vi "field raster.vi"(0 "field size":dbl, 2 "field number":u32) -> (10 "Plot1":cluster{dbl[], dbl[]}, 11 "Plot2":cluster{dbl[], dbl[]}, 14 "current X":dbl, 15 "current Y":dbl, 17 "x mark":dbl[](array[numeric]), 18 "y mark":dbl[](array[numeric]))   [LabVIEW 2014]
uses:
  stage-controller-globals.vi
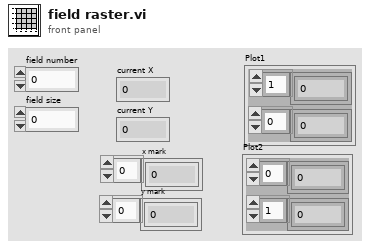
[diagram p1: front panel]
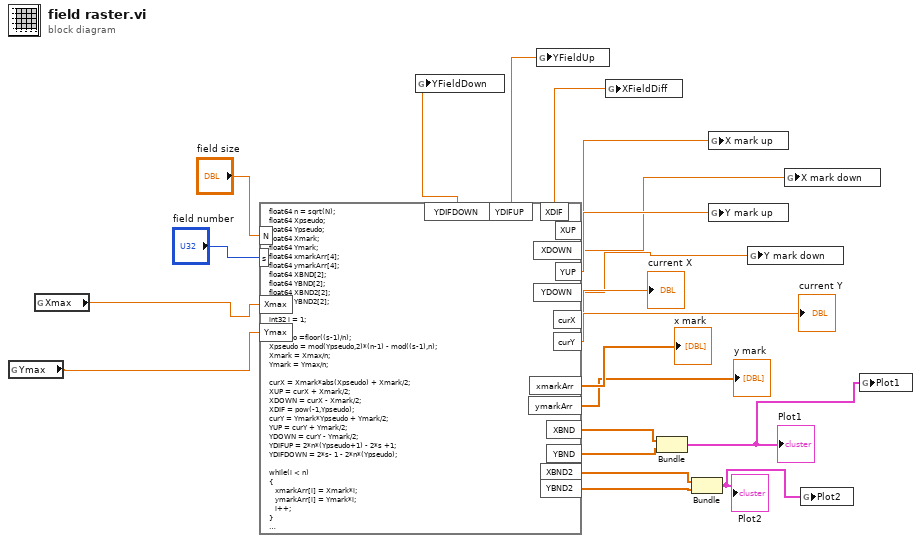
[diagram p0: block diagram]
diagram:
  n1 = global read "stage-controller-globals.vi" "Ymax"() -> (w10:dbl)
  n2 = global read "stage-controller-globals.vi" "Xmax"() -> (w11:dbl)
  n3 = formula code="float64 n = sqrt(N);\nfloat64 Xpseudo;\nfloat64 Ypseudo;\nfloat64 Xmark;\nfloat64 Ymark;\nfloat64 xmarkArr[4];\nfloat64 ymarkArr[4];\nfloat64 XBND[2];\nfloat64 YBND[2];\nfloat64 XBND2[2];\nfloat64 YBND2[2];\n\nint32 i = 1;\n\nYpseudo =floor((s-1)/n); \nXpseudo = mod(Ypseudo,2)*(n-1) - mod((s-1),n);\nXmark = Xmax/n;\nYmark = Ymax/n;\n\ncurX = Xmark*abs(Xpseudo) + Xmark/2;\nXUP = curX + Xmark/2;\nXDOWN = curX - Xmark/2;\nXDIF = pow(-1,Ypseudo);\ncurY = Ymark*Ypseudo + Ymark/2;\nYUP = curY + Ymark/2;\nYDOWN = curY - Ymark/2;\nYDIFUP = 2*n*(Ypseudo+1) - 2*s +1;\nYDIFDOWN = 2*s- 1 - 2*n*(Ypseudo);\n\nwhile(i < n)\n{\n   xmarkArr[i] = Xmark*i;\n   ymarkArr[i] = Ymark*i;\n   i++;\n}\n\ni = 0;\n\n XBND[i] = curX - Xmark/2;\nYBND[i] = curY - Ymark/2;\n i++;\nXBND[i] = curX + Xmark/2;\nYBND[i] = curY - Ymark/2;\n\ni=0;\n\nXBND2[i] = curX - Xmark/2;\nYBND2[i] =  curY + Ymark/2;\ni++;\nXBND2[i] = curX + Xmark/2;\nYBND2[i] =  curY + Ymark/2;\ni++;"("N"="field size", "s"="field number", "Xmax"=w11, "Ymax"=w10) -> ("curX"=→"current X":dbl, "curY"=→"current Y":dbl, "ymarkArr"=→"y mark":dbl[], "xmarkArr"=→"x mark":dbl[], "XUP"=w6:dbl, "YUP"=w7:dbl, "XBND"=w15:dbl[], "YBND"=w14:dbl[], "XBND2"=w13:dbl[], "YBND2"=w12:dbl[], "XDOWN"=w5:dbl, "YDOWN"=w4:dbl, "YDIFUP"=w3:dbl, "XDIF"=w2:dbl, "YDIFDOWN"=w1:dbl)
  n4 = global write "stage-controller-globals.vi" "YFieldDown"(w1) -> ()
  n5 = global write "stage-controller-globals.vi" "YFieldUp"(w3) -> ()
  n6 = global write "stage-controller-globals.vi" "XFieldDiff"(w2) -> ()
  n7 = Bundle(w15, w14) -> (w17:cluster{dbl[], dbl[]})  [unwired: 1 out]
  "Plot1" <- w17
  n8 = Bundle(w13, w12) -> (w16:cluster{dbl[], dbl[]})  [unwired: 1 out]
  "Plot2" <- w16
  n9 = global write "stage-controller-globals.vi" "X mark up"(w6) -> ()
  n10 = global write "stage-controller-globals.vi" "Y mark up"(w7) -> ()
  n11 = global write "stage-controller-globals.vi" "Y mark down"(w4) -> ()
  n12 = global write "stage-controller-globals.vi" "X mark down"(w5) -> ()
  n13 = global write "stage-controller-globals.vi" "Plot2"(w16) -> ()
  n14 = global write "stage-controller-globals.vi" "Plot1"(w17) -> ()
